vi "sv_Compute High Pass Filter Denominator.vi"(0 "wn":dbl, 7 "s":cdb, 11 "Q1":dbl=0.7071067811865475 format="%#_26g") -> (4 "result":cdb)   [LabVIEW 2017]
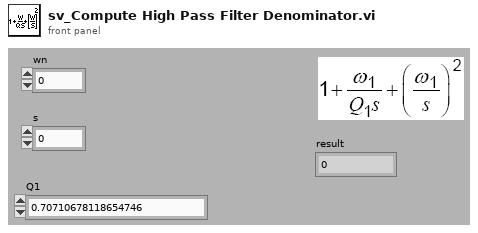
[diagram p1: front panel]
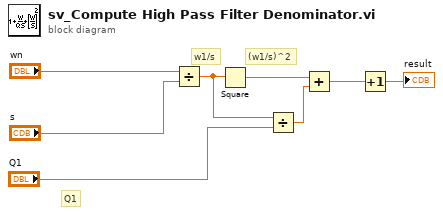
[diagram p0: block diagram]
diagram:
  # "(w1/s)^2"
  # "w1/s"
  # "Q1"
  n1 = Divide(x="wn", y="s") -> (x/y=w6:cdb)
  n2 = Square(x=w6) -> (x^2=w7:cdb)
  n3 = Divide(x=w6, y="Q1") -> (x/y=w8:cdb)
  n4 = Add(x=w7, y=w8) -> (x+y=w3:cdb)
  n5 = Increment(x=w3) -> (x+1=→"result":cdb)
